vi "Handle Drag Over.vi"(8 "error in (no error)":errorcluster, 10 "Coords":T1, 11 "Process Builder View in":refnum<class "Process Builder View.lvclass">) -> (0 "error out":errorcluster, 2 "Discard?":bool, 3 "Process Builder View out":refnum<class "Process Builder View.lvclass">)   [LabVIEW 2019, in "Process Builder View.lvclass"]
uses:
  <vilib>/gpm_packages/@cs/Car-wash/Source/Process Builder View/Process Builder View.lvclass
  <vilib>/Utility/miscctls.llb/LVPoint32TypeDef.ctl
  <vilib>/gpm_packages/@cs/Test-executive-builder/Source/Test Executive Builder View/Test Executive Builder View/Test Executive Builder View.lvclass
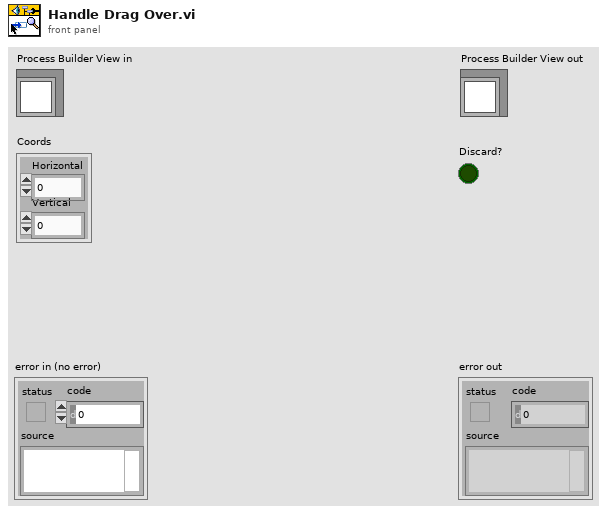
[diagram p1: front panel]
types:
  T1 = typedef "LVPoint32TypeDef.ctl" = cluster{"Horizontal":i32, "Vertical":i32}
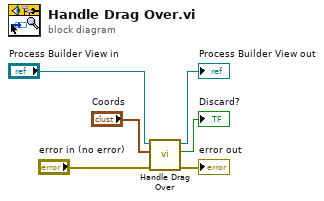
[diagram p0: block diagram]
diagram:
  n1 = call-parent "Handle Drag Over.vi"("error in (no error)"="error in (no error)", "Coords"="Coords", "Test Executive Builder View in"="Process Builder View in") -> ("error out"=→"error out":errorcluster, "Discard?"=→"Discard?":bool, "Test Executive Builder View out"=→"Process Builder View out":refnum<class "Process Builder View.lvclass">)  [unwired: 6 in]
